vi "SetParameter.vi"(8 "error in (no error)":errorcluster, 10 "SetParameter":T1, 11 "PacificPowerSource in":refnum<class "PacificPowerSource.lvclass">) -> (0 "error out":errorcluster, 2 "StatusUpdates":string[](array[string]), 3 "PacificPowerSource out":refnum<class "PacificPowerSource.lvclass">)   [LabVIEW 2018, in "AcPwrPlugins.lvlib" / "PacificPowerSource.lvclass"]
uses:
  PacificPowerSource.lvclass
  AcPwrBaseClass/TypeDefs/SetParameterInputs.ctl
  AcPwrBaseClass/AcPwrBase.lvclass
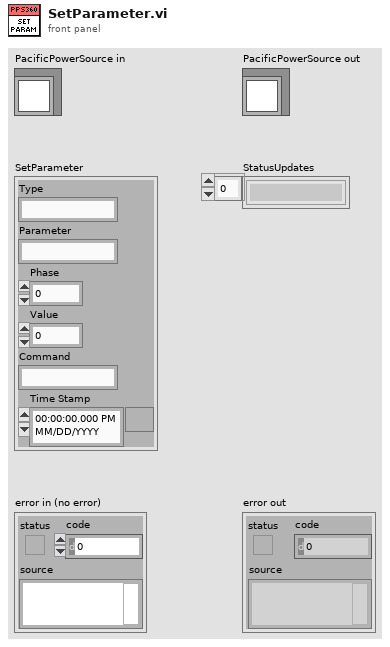
[diagram p1: front panel]
types:
  T1 = typedef "AcPwrPlugins.lvlib/AcPwrBase.lvclass/SetParameterInputs.ctl" = cluster{"Type":string, "Parameter":string, "Phase":i32, "Value":dbl, "Command":string, "Time Stamp":timestamp}
  T2 = typedef "AcPwrPlugins.lvlib/PacificPowerSource.lvclass/Modules.ctl" = cluster{"Handle":string, "Connected":bool, "Clear Device (F)":bool, "btnIdQuery":bool, "btnReset":bool, "Program #":cluster{"Phase B (Degrees)":i32, "Waveform A (1: Sine)":i32, "Voltage Level (Va)":dbl, "Program Number (0)":i32, "Voltage Level (Vb) ":dbl, "Form (3: Three)":u16, "Coupling  (0: Direct)":u16, "Frequency (45Hz)":dbl, "Current Limit (40A)":dbl, "Phase C (Degrees)":i32, "Voltage Level (Vc)":dbl, "Waveform B (1: Sine)":i32, "Waveform C (1: Sine)":i32}[], "Impedance Parameters (off, 0.00)":cluster{"State":bool, "Impedance":dbl}, "Transient Execution (F)":bool, "OutputEnabled":bool, "Source Range":cluster{"Frequency Minimum (45 Hz)":dbl, "Frequency Maximum (1200 Hz)":dbl, "Voltage Maximum (V)":dbl, "Voltage Minimum (V)":dbl, "Range Control (0: Auto)":u16, "Initial Voltage (0V)":u16, "Frequency Range (600Hz)":u16}, "Port Type":enum16{"GPIB", "Serial"}}[]
  T3 = cluster{"Handle":string, "Connected":bool, "Clear Device (F)":bool, "btnIdQuery":bool, "btnReset":bool, "Program #":cluster{"Phase B (Degrees)":i32, "Waveform A (1: Sine)":i32, "Voltage Level (Va)":dbl, "Program Number (0)":i32, "Voltage Level (Vb) ":dbl, "Form (3: Three)":u16, "Coupling  (0: Direct)":u16, "Frequency (45Hz)":dbl, "Current Limit (40A)":dbl, "Phase C (Degrees)":i32, "Voltage Level (Vc)":dbl, "Waveform B (1: Sine)":i32, "Waveform C (1: Sine)":i32}[], "Impedance Parameters (off, 0.00)":cluster{"State":bool, "Impedance":dbl}, "Transient Execution (F)":bool, "OutputEnabled":bool, "Source Range":cluster{"Frequency Minimum (45 Hz)":dbl, "Frequency Maximum (1200 Hz)":dbl, "Voltage Maximum (V)":dbl, "Voltage Minimum (V)":dbl, "Range Control (0: Auto)":u16, "Initial Voltage (0V)":u16, "Frequency Range (600Hz)":u16}, "Port Type":enum16{"GPIB", "Serial"}}
  T4 = cluster{"Handle":string, "Connected":bool, "Clear Device (F)":bool, "btnIdQuery":bool, "btnReset":bool, "Program #":cluster{"Phase B (Degrees)":i32, "Waveform A (1: Sine)":i32, "Voltage Level (Va)":dbl, "Program Number (0)":i32, "Voltage Level (Vb) ":dbl, "Form (3: Three)":u16, "Coupling  (0: Direct)":u16, "Frequency (45Hz)":dbl, "Current Limit (40A)":dbl, "Phase C (Degrees)":i32, "Voltage Level (Vc)":dbl, "Waveform B (1: Sine)":i32, "Waveform C (1: Sine)":i32}[], "Impedance Parameters (off, 0.00)":cluster{"State":bool, "Impedance":dbl}, "Transient Execution (F)":bool, "OutputEnabled":bool, "Source Range":cluster{"Frequency Minimum (45 Hz)":dbl, "Frequency Maximum (1200 Hz)":dbl, "Voltage Maximum (V)":dbl, "Voltage Minimum (V)":dbl, "Range Control (0: Auto)":u16, "Initial Voltage (0V)":u16, "Frequency Range (600Hz)":u16}, "Port Type":enum16{"GPIB", "Serial"}}[]
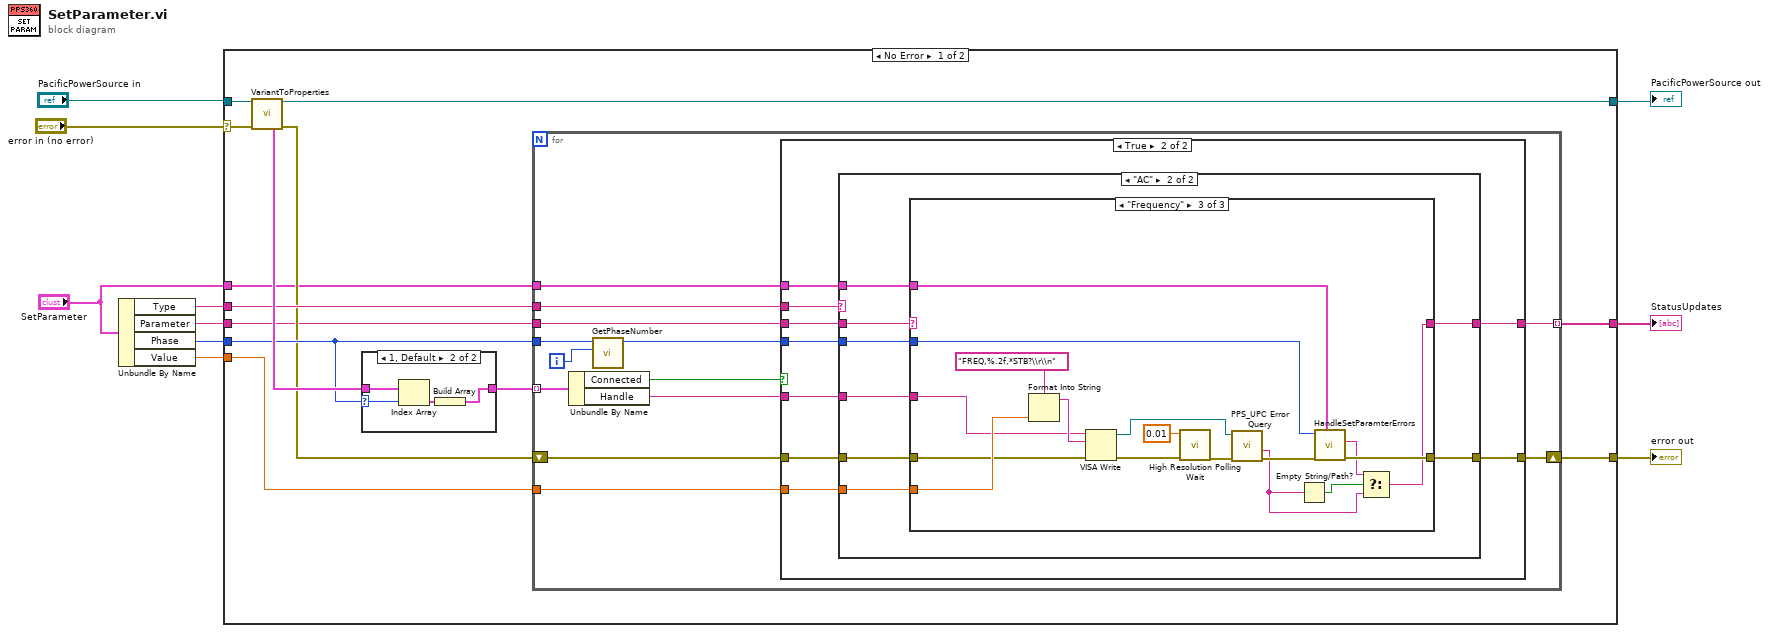
[diagram p0: block diagram]
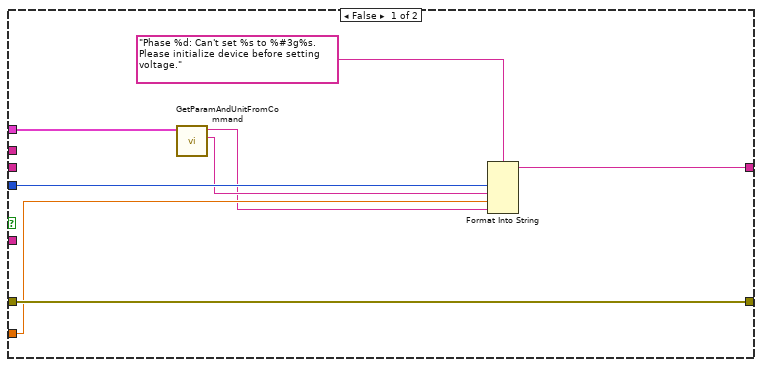
[diagram p3: hidden frame]
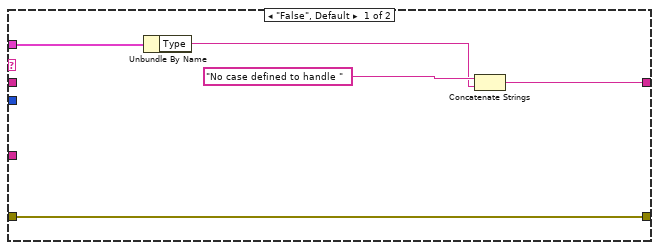
[diagram p4: hidden frame]
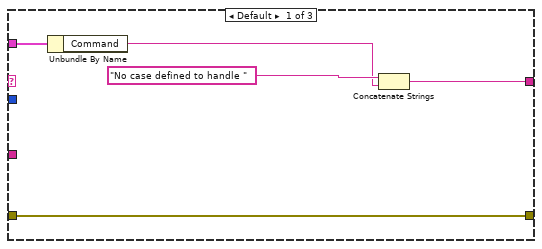
[diagram p5: hidden frame]
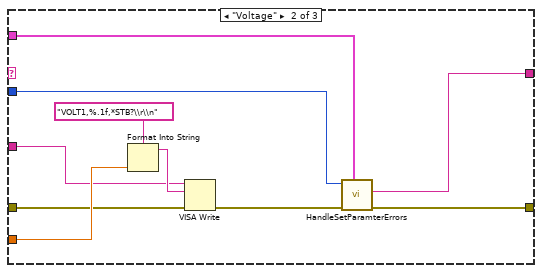
[diagram p6: hidden frame]
diagram:
  n1 = Unbundle By Name("SetParameter") -> ("Type"=w8:string, "Parameter"=w7:string, "Phase"=w10:i32, "Value"=w9:dbl)
  n2 = case shown="No Error" "error in (no error)" {
    selector: "error in (no error)" -> [w16 w105]
    tunnel: "PacificPowerSource in" -> [w23 w104]
    tunnel: [w22 w104] -> w5
    tunnel: w10 -> [w19 _]
    tunnel: [w18 _] -> w1
    tunnel: w8 -> [w17 _]
    tunnel: [w14 w105] -> w2
    tunnel: w9 -> [w13 _]
    tunnel: w7 -> [w12 _]
    tunnel: "SetParameter" -> [w11 _]
    frame No Error {
      n3 = call "VariantToProperties.vi"("PacificPowerSource in"=w23, "error in (no error)"=w16) -> ("PacificPowerSource out"=w22:refnum<class "PacificPowerSource.lvclass">, "Modules"=w21:T2, "error out"=w15:errorcluster)  [unwired: 7 in, 4 out]
      n4 = case shown="1, Default" w19 {
        selector: w19 -> [_ w25]
        tunnel: w21 -> [w24 w28]
        tunnel: [w24 w26] -> w20
        frame -1 {
        }
        frame 1, Default {
          n5 = Index Array(array=w28, index=w25) -> (element=w27:T3)
          n6 = Build Array(w27) -> (w26:T4)
        }
      }
      n7 = for {
        tunnel: w20 -> [w41] mode=indexing
        shift-right: [w39] -> w14
        shift-left: w15 -> [w40]
        tunnel: w13 -> [w36]
        tunnel: w19 -> [w34]
        tunnel: [w32] -> w18 mode=indexing
        tunnel: w17 -> [w31]
        tunnel: w12 -> [w30]
        tunnel: w11 -> [w29]
        i -> [w35]
        n8 = Unbundle By Name(w41) -> ("Connected"=w38:bool, "Handle"=w37:string)
        n9 = call "GetPhaseNumber.vi"("Loop Counter"=w35, "Phase(-1, all) in"=w34) -> ("Phase(-1, all) out"=w33:i32)  [unwired: 9 in]
        n10 = case shown="True" w38 {
          tunnel: w40 -> [w49 w58]
          tunnel: [w49 w57] -> w39
          tunnel: w37 -> [_ w56]
          tunnel: w36 -> [w43 w55]
          tunnel: w33 -> [w48 w54]
          tunnel: [w46 w53] -> w32
          tunnel: w31 -> [_ w52]
          tunnel: w30 -> [_ w51]
          tunnel: w29 -> [w45 w50]
          frame False {
            n11 = call "GetParamAndUnitFromCommand.vi"("SetParameter"=w45) -> ("Parameter"=w44:string, "Unit Label"=w42:string)  [unwired: 9 in]
            n12 = Format Into String(format string="Phase %d: Can't set %s to %#3g%s. Please initialize device before setting voltage.", w48, w44, w43, w42) -> (resulting string=w46:string)  [unwired: 2 in, 1 out]
          }
          frame True {
            n13 = case shown="\"AC\"" w52 {
              tunnel: w58 -> [w59 w71]
              tunnel: [w59 w70] -> w57
              tunnel: w56 -> [_ w69]
              tunnel: w55 -> [_ w68]
              tunnel: w54 -> [_ w67]
              tunnel: [w60 w66] -> w53
              tunnel: w51 -> [_ w65]
              tunnel: w50 -> [w61 w64]
              frame "False", Default {
                n14 = Unbundle By Name(w61) -> ("Type"=w62:string)
                n15 = Concatenate Strings("No case defined to handle " ("string"), w62) -> (w60:string)
              }
              frame "AC" {
                n16 = case shown="\"Frequency\"" w65 {
                  tunnel: w71 -> [w76 w78 w96]
                  tunnel: [w76 w86 w103] -> w70
                  tunnel: w69 -> [_ w79 w97]
                  tunnel: w68 -> [_ w81 w99]
                  tunnel: w67 -> [_ w85 w102]
                  tunnel: [w75 w84 w91] -> w66
                  tunnel: w64 -> [w73 w83 w101]
                  frame Default {
                    n17 = Unbundle By Name(w73) -> ("Command"=w72:string)
                    n18 = Concatenate Strings("No case defined to handle " ("string"), w72) -> (w75:string)
                  }
                  frame "Voltage" {
                    n19 = Format Into String(format string="VOLT1,%.1f,*STB?\\r\\n", w81) -> (resulting string=w80:string)  [unwired: 2 in, 1 out]
                    n20 = VISA Write(VISA resource name=w79, write buffer=w80, error in (no error)=w78) -> (error out=w77:errorcluster)  [unwired: 2 out]
                    n21 = call "HandleSetParamterErrors.vi"("SetParameter"=w83, "error in (no error)"=w77, "Phase"=w85) -> ("error IO"=w86:errorcluster, "Status Update"=w84:string)  [unwired: 7 in]
                  }
                  frame "Frequency" {
                    n22 = Format Into String(format string="FREQ,%.2f,*STB?\\r\\n", w99) -> (resulting string=w98:string)  [unwired: 2 in, 1 out]
                    n23 = VISA Write(VISA resource name=w97, write buffer=w98, error in (no error)=w96) -> (VISA resource name out=w88:refnum<visa-resource-name>, error out=w95:errorcluster)  [unwired: 1 out]
                    n24 = call <vilib>:"High Resolution Polling Wait.vi"("error in (no error)"=w95, "seconds to wait"=0.01) -> ("error out"=w90:errorcluster)  [unwired: 9 in]
                    n25 = call <instrlib>:"PPS_UPC Error Query.vi"("error in (no error)"=w90, "VISA session"=w88) -> ("error out"=w89:errorcluster, "Error Message"=w87:string)  [unwired: 6 in, 2 out]
                    n26 = Empty String/Path?(string/path=w87) -> (empty?=w93:bool)
                    n27 = call "HandleSetParamterErrors.vi"("SetParameter"=w101, "error in (no error)"=w89, "Phase"=w102) -> ("error IO"=w103:errorcluster, "Status Update"=w92:string)  [unwired: 7 in]
                    n28 = Select(t=w92, s=w93, f=w87) -> (s? t:f=w91:string)
                  }
                }
              }
            }
          }
        }
      }
    }
    frame Error {
    }
  }
  "error out" <- w2
  "PacificPowerSource out" <- w5
  "StatusUpdates" <- w1
